vi "Get_Trend Data.vi"(7 "LabVIEW Web Service Request":refnum<class "Web Request.lvclass">) -> (3 "trendData":string)   [LabVIEW 2016]
uses:
  <vilib>/wsapi/Web Request.lvclass
  Store Data/Data Library.lvlib
panel:
  # "Use the Web Service Request input terminal to call the VIs on the Web Services palette. Do not remove it from the connector pane unless you don't need access to the palette."
  # "Each additional control wired to the connector pane will be available as an input in the URL. To include an indicator in terminal-mode output (the default setting), it must also be wired to the connector pane."
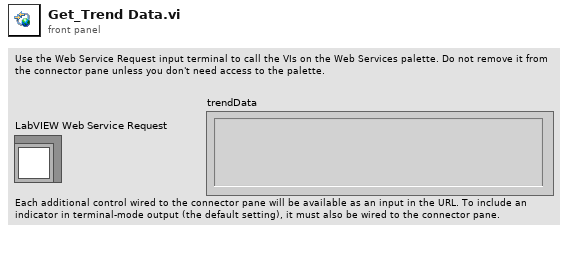
[diagram p1: front panel]
types:
  T1 = enum16{"Create", "Enqueue", "Preview Data", "Destroy"}
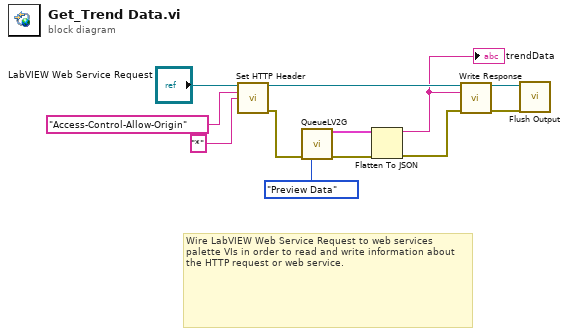
[diagram p0: block diagram]
diagram:
  # "Wire LabVIEW Web Service Request to web services palette VIs in order to read and write information about the HTTP request or web service."
  n1 = call <vilib>:"Set HTTP Header.vi"("LabVIEW Web Service Request"="LabVIEW Web Service Request", "header"="Access-Control-Allow-Origin", "header value"="*") -> ("LabVIEW Web Service Request out"=w7:refnum<class "Web Request.lvclass">, "error out"=w3:errorcluster)  [unwired: 11 in]
  n2 = call "QueueLV2G.vi"("error in (no error)"=w3, "Selector"=T1."Preview Data") -> ("r[]"=w5:cluster{"h":dbl, "l":dbl, "c":dbl, "s":bool}[], "error out"=w2:errorcluster)  [unwired: 12 in]
  n3 = Flatten To JSON(anything=w5, error in (no error)=w2) -> (JSON string=w4:string, 11:w1:errorcluster)  [unwired: 1 in]
  "trendData" <- w4
  n4 = call <vilib>:"Write Response.vi"("LabVIEW Web Service Request"=w7, "response string"=w4, "error in (no error)"=w1) -> ("LabVIEW Web Service Request out"=w11:refnum<class "Web Request.lvclass">, "error out"=w10:errorcluster)  [unwired: 11 in]
  n5 = call <vilib>:"Flush Output.vi"("LabVIEW Web Service Request"=w11, "error in (no error)"=w10) -> ()  [unwired: 12 in, 2 out]
